vi "Sub_Zerofill.vi"(11 "数値":i32) -> (3 "結果文字列":string)   [LabVIEW 2018]
panel:
  # "<機能>\n　数値を0右埋めの文字列にする"
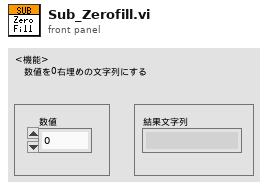
[diagram p1: front panel]
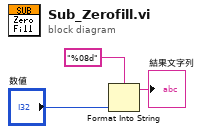
[diagram p0: block diagram]
diagram:
  n1 = Format Into String(format string="%08d" ("形式文字列"), "数値") -> (resulting string=→"結果文字列":string)  [unwired: 2 in, 1 out]
